vi "Phasor Compute Calibrated Phasor Array.vi"(6 "Phasor Calibration Data":T7, 7 "Phasor Calculation":T1, 8 "Error In":errorcluster, 9 "Gates Definitions":T4={"First Gate: t1"=0.0, "Gate Width: W"=0.0, "Gate Step: d"=0.0, "# Gates: G"=0.0, "Use Gate Center"=FALSE, "Frames/Image: F"=50, "Gates/Frame: L"=0, "Bits/Frame: q"=0, "Multiplicity: p"=0, "Gate Type"=enum."Square", "Gate Edge s"=4.0, "Gate Top Slope"=4.0, "Reversed Sawtooth?"=FALSE, "Computation"=FALSE, "User-defined Gate"={"X Array"=[], "Y Array"=[]}, "Tolerance"=50.0, "Integration"=enum."Item 0", "# Steps"=50.0, "Type of User-defined Function"=enum."Gate"}, 10 "Decay Definition":T2={"offset: t0"=0.0, "period: T"=0.0, "lifetime: tau"=0.0, "Incident Signal: I"=0.5, "Normalized Decays"=FALSE, "IRF Model"=enum."Dirac", "IRF Parameter 1"=0.0, "Poisson Signal"=FALSE}, 11 "Lifetime Array":ext[](array[numeric])) -> (0 "Error Out":errorcluster, 1 "Calibrated s Array":ext[](array[numeric]), 2 "Calibrated g Array":ext[](array[numeric]), 3 "True Lifetime Array":ext[](array[numeric]), 4 "# Rejected Pairs":i32, 5 "CPU (s)":dbl)   [LabVIEW 2021, in "Phasor.lvlib"]
uses:
  Phasor.lvlib
  Phasor Calibration Data.ctl
  Phasor Gate Definitions.ctl
  Phasor Gate Type.ctl
  Graphs/XY Graph/XY Plot Data.ctl
  Phasor Decay Definiton.ctl
  Phasor IRF Model.ctl
  Phasor Calculation Type.ctl
  Phasor Abort Parallel Computation.vi
  <vilib>/Utility/error.llb/Error Cluster From Error Code.vi
  <vilib>/ErrorRing/Error Ring.xnode
  Utilities/Utilities.lvlib
  Graphs/XY Graph/XY Graph Add-Ons.lvlib
panel:
  out "Uncalibrated Phasors":cxt[](array[numeric])
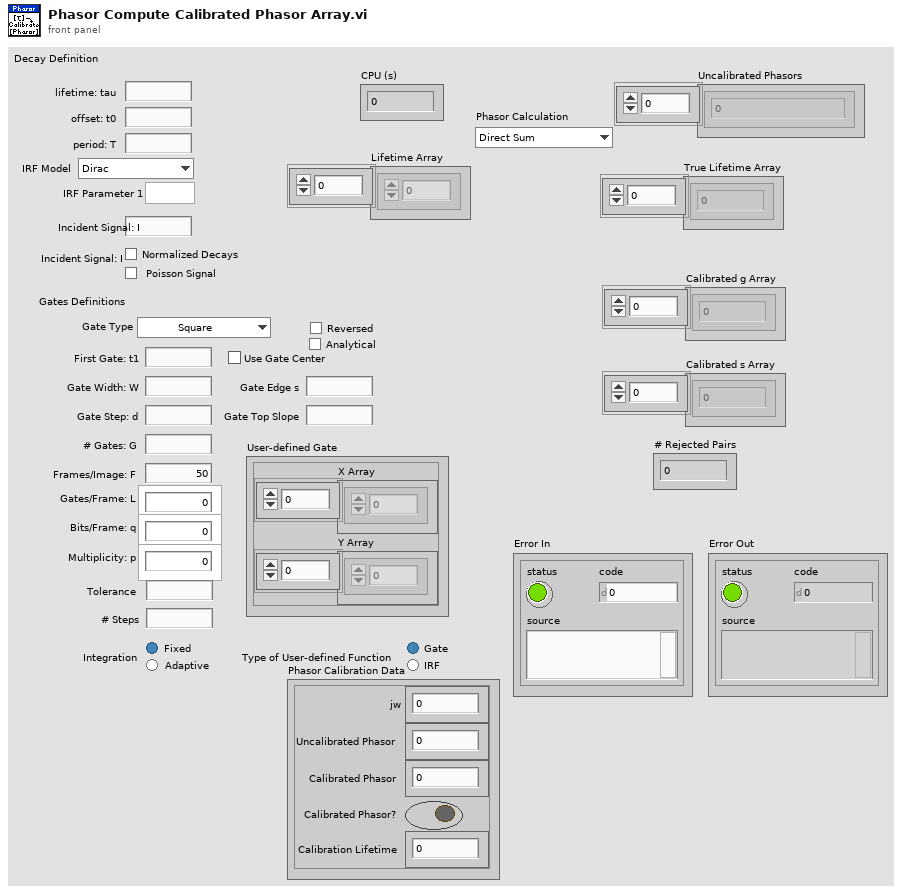
[diagram p1: front panel]
types:
  T1 = typedef "Phasor.lvlib/Phasor Calculation Type.ctl" = enum16{"Direct Sum", "Analytical Formula"}
  T2 = typedef "Phasor.lvlib/Phasor Decay Definiton.ctl" = cluster{"offset: t0":ext, "period: T":ext, "lifetime: tau":ext, "Incident Signal: I":ext, "Normalized Decays":bool, "IRF Model":T3, "IRF Parameter 1":ext, "Poisson Signal":bool}
  T3 = typedef "Phasor.lvlib/Phasor IRF Model.ctl" = enum16{"Dirac", "Exponential"}
  T4 = typedef "Phasor.lvlib/Phasor Gate Definitions.ctl" = cluster{"First Gate: t1":ext, "Gate Width: W":ext, "Gate Step: d":ext, "# Gates: G":ext, "Use Gate Center":bool, "Frames/Image: F":i32, "Gates/Frame: L":i32, "Bits/Frame: q":i32, "Multiplicity: p":i32, "Gate Type":T5, "Gate Edge s":ext, "Gate Top Slope":ext, "Reversed Sawtooth?":bool, "Computation":bool, "User-defined Gate":T6, "Tolerance":ext, "Integration":enum32{"Item 0", "Item 1"}, "# Steps":ext, "Type of User-defined Function":enum32{"Gate", "IRF"}}
  T5 = typedef "Phasor.lvlib/Phasor Gate Type.ctl" = enum16{"Square", "Finite Edge Square", "Finite Edge, Tilted Top Square", "Triangle", "Sawtooth", "User-defined"}
  T6 = typedef "XY Graph Add-Ons.lvlib/XY Plot Data.ctl" = cluster{"X Array":dbl[], "Y Array":dbl[]}
  T7 = typedef "Phasor.lvlib/Phasor Calibration Data.ctl" = cluster{"jw":cxt, "Uncalibrated Phasor":cxt, "Calibrated Phasor":cxt, "Calibrated Phasor?":bool, "Calibration Lifetime":ext}
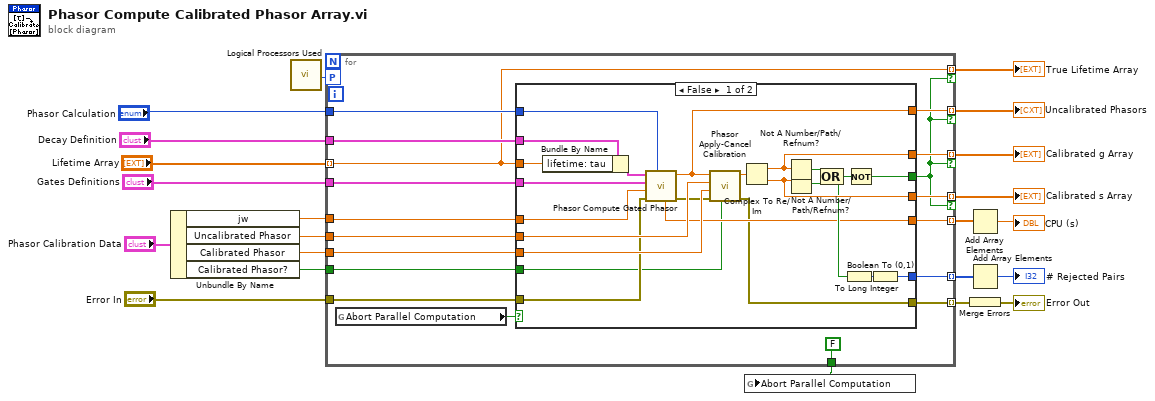
[diagram p0: block diagram]
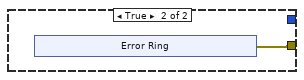
[diagram p2: hidden frame]
diagram:
  n1 = Unbundle By Name("Phasor Calibration Data") -> ("jw"=w19:cxt, "Uncalibrated Phasor"=w20:cxt, "Calibrated Phasor"=w21:cxt, "Calibrated Phasor?"=w22:bool)
  n2 = call "Logical Processors Used.vi"() -> ("# Logical Processor Used"=w1:i32)  [unwired: 6 in]
  n3 = for {
    tunnel: "Lifetime Array" -> [w23] mode=indexing
    tunnel: w19 -> [w40]
    tunnel: [w33] -> w13 mode=indexing if=w30
    tunnel: [w32] -> w14 mode=indexing if=w30
    tunnel: "Gates Definitions" -> [w39]
    tunnel: "Decay Definition" -> [w38]
    tunnel: w20 -> [w37]
    tunnel: w21 -> [w36]
    tunnel: w22 -> [w27]
    tunnel: "Phasor Calculation" -> [w35]
    tunnel: [w23] -> w9 mode=indexing if=w30
    tunnel: [w31] -> w8 mode=indexing if=w30
    tunnel: "Error In" -> [w34]
    tunnel: [w26] -> w10 mode=indexing
    tunnel: [w29] -> w6 mode=indexing
    tunnel: [w28] -> w4 mode=indexing
    workers-P: w1 -> [_]
    tunnel: [FALSE ("Abort Parallel Computation")] -> w2
    n4 = global read "Phasor Abort Parallel Computation.vi" "Abort Parallel Computation"() -> (w24:bool)
    n5 = case shown="False" w24 {
      tunnel: w40 -> [w62 _]
      tunnel: w39 -> [w61 _]
      tunnel: w38 -> [w60 _]
      tunnel: w37 -> [w58 _]
      tunnel: w36 -> [w57 _]
      tunnel: w35 -> [w56 _]
      tunnel: w34 -> [w55 _]
      tunnel: [w54 _] -> w33
      tunnel: [w53 _] -> w32
      tunnel: w23 -> [w50 _]
      tunnel: [w49 _] -> w31
      tunnel: [w48 _] -> w30
      tunnel: [w45 _] -> w29
      tunnel: [w44 _] -> w28
      tunnel: w27 -> [w43 _]
      tunnel: [w41 w64] -> w26
      frame False {
        n6 = Bundle By Name(cluster=w60, "lifetime: tau"=w50) -> (w63:T2)
        n7 = call "Phasor Compute Gated Phasor.vi"("Phasor Calculation Type"=w56, "Error In"=w55, "j 2 pi f"=w62, "Gates Definitions"=w61, "Decay Definition"=w63) -> ("Error Out"=w42:errorcluster, "phasor"=w49:cxt, "CPU (s)"=w44:dbl)  [unwired: 4 in]
        n8 = call "Phasor Apply-Cancel Calibration.vi"("Calibrated Phasor"=w43, "Error In"=w42, "Target Phasor"=w57, "Calibration Phasor"=w58, "Phasor in"=w49) -> ("Error Out"=w41:errorcluster, "Phasor out"=w59:cxt)  [unwired: 5 in]
        n9 = Complex To Re/Im(x + iy=w59) -> (x=w54:ext, y=w53:ext)
        n10 = Not A Number/Path/Refnum?(number/path/refnum=w54) -> (NaN/Path/Refnum?=w52:bool)
        n11 = Not A Number/Path/Refnum?(number/path/refnum=w53) -> (NaN/Path/Refnum?=w51:bool)
        n12 = Compound Arithmetic op=OR(w52, w51) -> (w47:bool)
        n13 = Boolean To (0,1)(Boolean=w47) -> (0, 1=w46:i16)
        n14 = Not(x=w47) -> (.not. x?=w48:bool)
        n15 = To Long Integer(number=w46) -> (32bit integer=w45:i32)
      }
      frame True {
        n16 = xnode "Error Ring"() -> ("error out"=w64:errorcluster)
      }
    }
  }
  "Calibrated s Array" <- w14
  "Calibrated g Array" <- w13
  "True Lifetime Array" <- w9
  "Uncalibrated Phasors" <- w8
  n17 = global write "Phasor Abort Parallel Computation.vi" "Abort Parallel Computation"(w2) -> ()
  n18 = Add Array Elements(numeric array=w4) -> (sum=→"CPU (s)":dbl)
  n19 = Add Array Elements(numeric array=w6) -> (sum=→"# Rejected Pairs":i32)
  n20 = Merge Errors(w10) -> (→"Error Out":errorcluster)
